vi "ChordsRecognitionFinal.vi"() -> ()   [LabVIEW 2021]
uses:
  <vilib>/Utility/NIReport.llb/Report Type.ctl
  <vilib>/numeric/Random Number (Range) I64.vi
  <vilib>/Analysis/baseanly.llb/Real A x B.vi
  <vilib>/numeric/sub_Random U32.vi
  <vilib>/Utility/file.llb/Read Delimited Spreadsheet (DBL).vi
  <vilib>/addons/_office/excel.llb/Excel Easy Table (str).vi
  <vilib>/Analysis/Matrix/Numeric/Conversions/Matrix To Array - RM.vi
  <vilib>/Utility/NIReport.llb/NI_report.lvclass
  <vilib>/Analysis/NI_AALBase.lvlib
  <vilib>/Analysis/Matrix/NI_Matrix.lvlib
  <vilib>/Utility/NIReport.llb/NI_ReportGenerationCore.lvlib
  <vilib>/Utility/NIReport.llb/Excel/NI_Excel.lvclass
  <vilib>/addons/_office/NI_ReportGenerationToolkit.lvlib
panel:
  in  "Save":bool
  in  "Init":bool
  in  "Aux":dbl
  in  "Saved":bool
  out "n":i32
  in  "Y_ideal":dbl[][][](array[numeric])
  out "Playing":string
  out "Keys":bool[][](array[boolean])
  out "la#":bool
  out "sol#":bool
  out "fa#":bool
  out "re#":bool
  out "do#":bool
  out "si":bool
  out "la":bool
  out "sol":bool
  out "fa":bool
  out "mi":bool
  out "re":bool
  out "do":bool
  out "Confidence":dbl
  out "min value":dbl
  out "max value":dbl
  in  "Init - Random":bool
  in  "Output":i32=1
  in  "2th layer":i32=2
  in  "1th layer":i32=3
  in  "Predict":bool
  out "Error":dbl[](array[numeric])
  in  "W1":dbl[][](array[numeric])
  out "Y":dbl[][](array[numeric])
  in  "Learn?":bool
  in  "Lr":dbl
  in  "?":bool
  in  "Bias 2":dbl[][](array[numeric]) format="%#_13g"
  in  "Bias 3":dbl[][](array[numeric]) format="%#_13g"
  in  "Bias 1":dbl[][](array[numeric]) format="%#_13g"
  in  "W2":dbl[][](array[numeric])
  in  "W3":dbl[][](array[numeric])
  out "C":i16[][](array[numeric])
  in  "index":i32
  out "BoolAux":bool[](array[boolean])
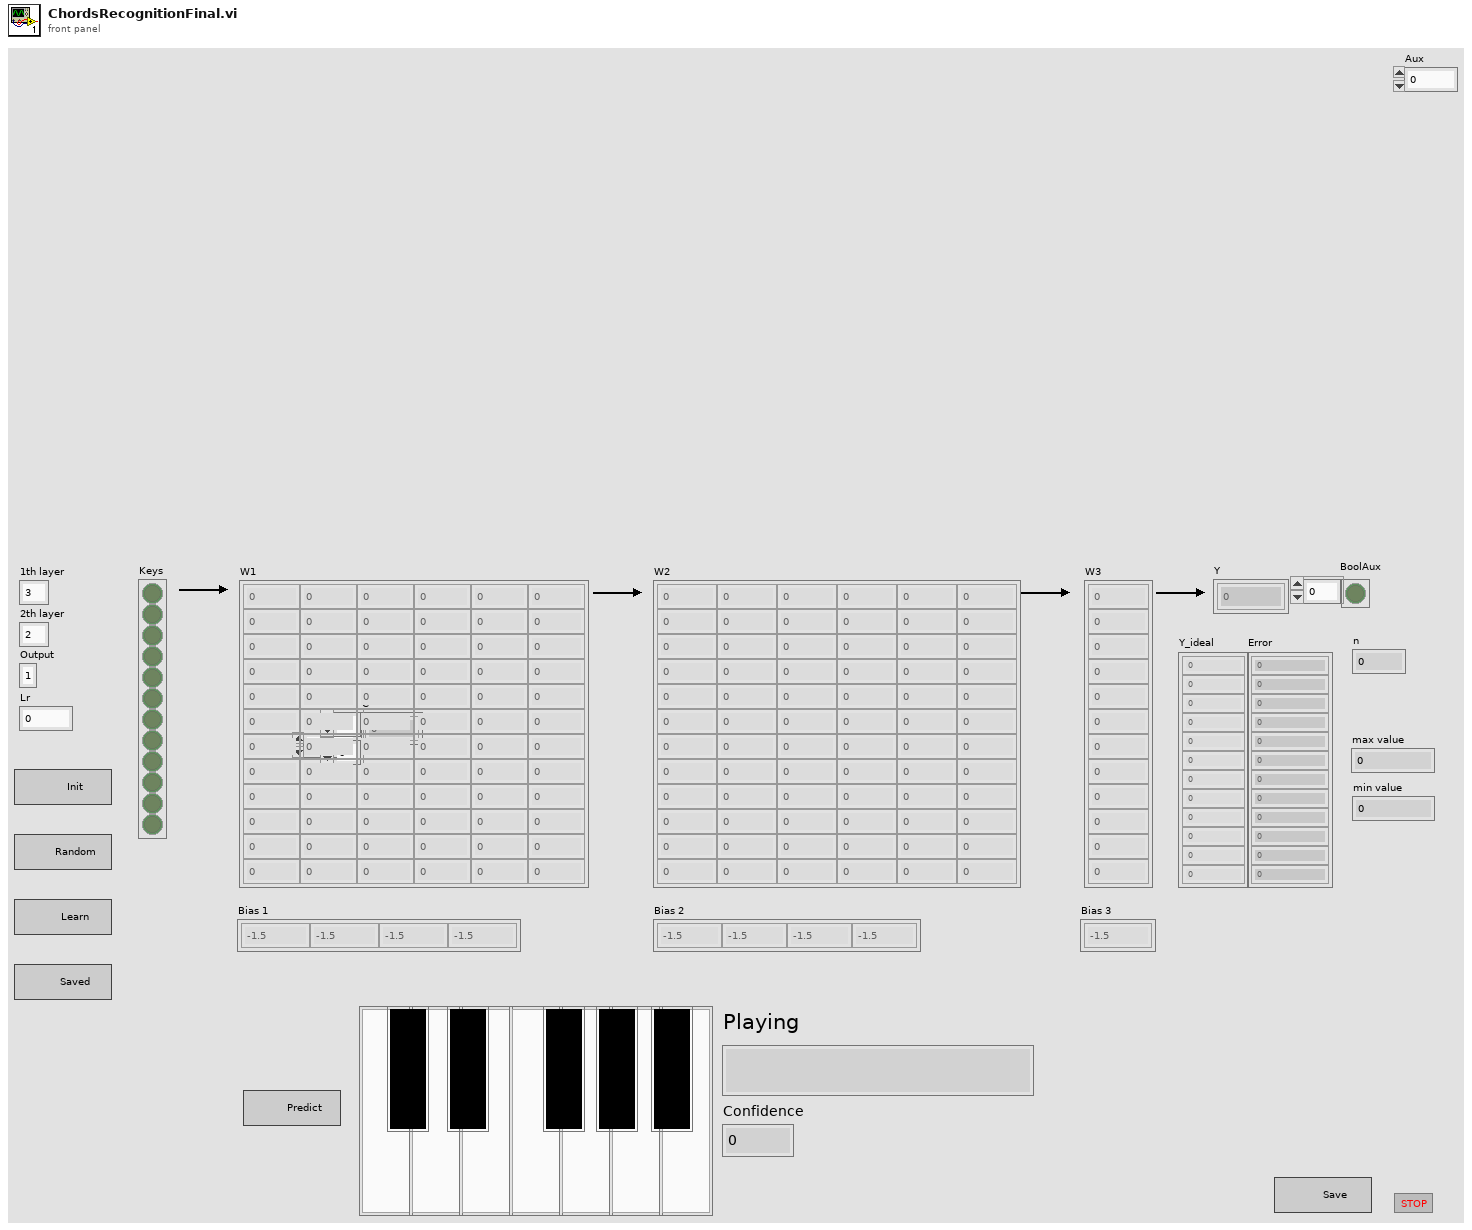
[diagram p1: front panel]
types:
  T1 = typedef "NI_ReportGenerationCore.lvlib/Report Type.ctl" = enum16{"HTML", "Word", "Excel"}
  T2 = typedef "NI_Matrix.lvlib/RealMatrix.ctl" = dbl[][]
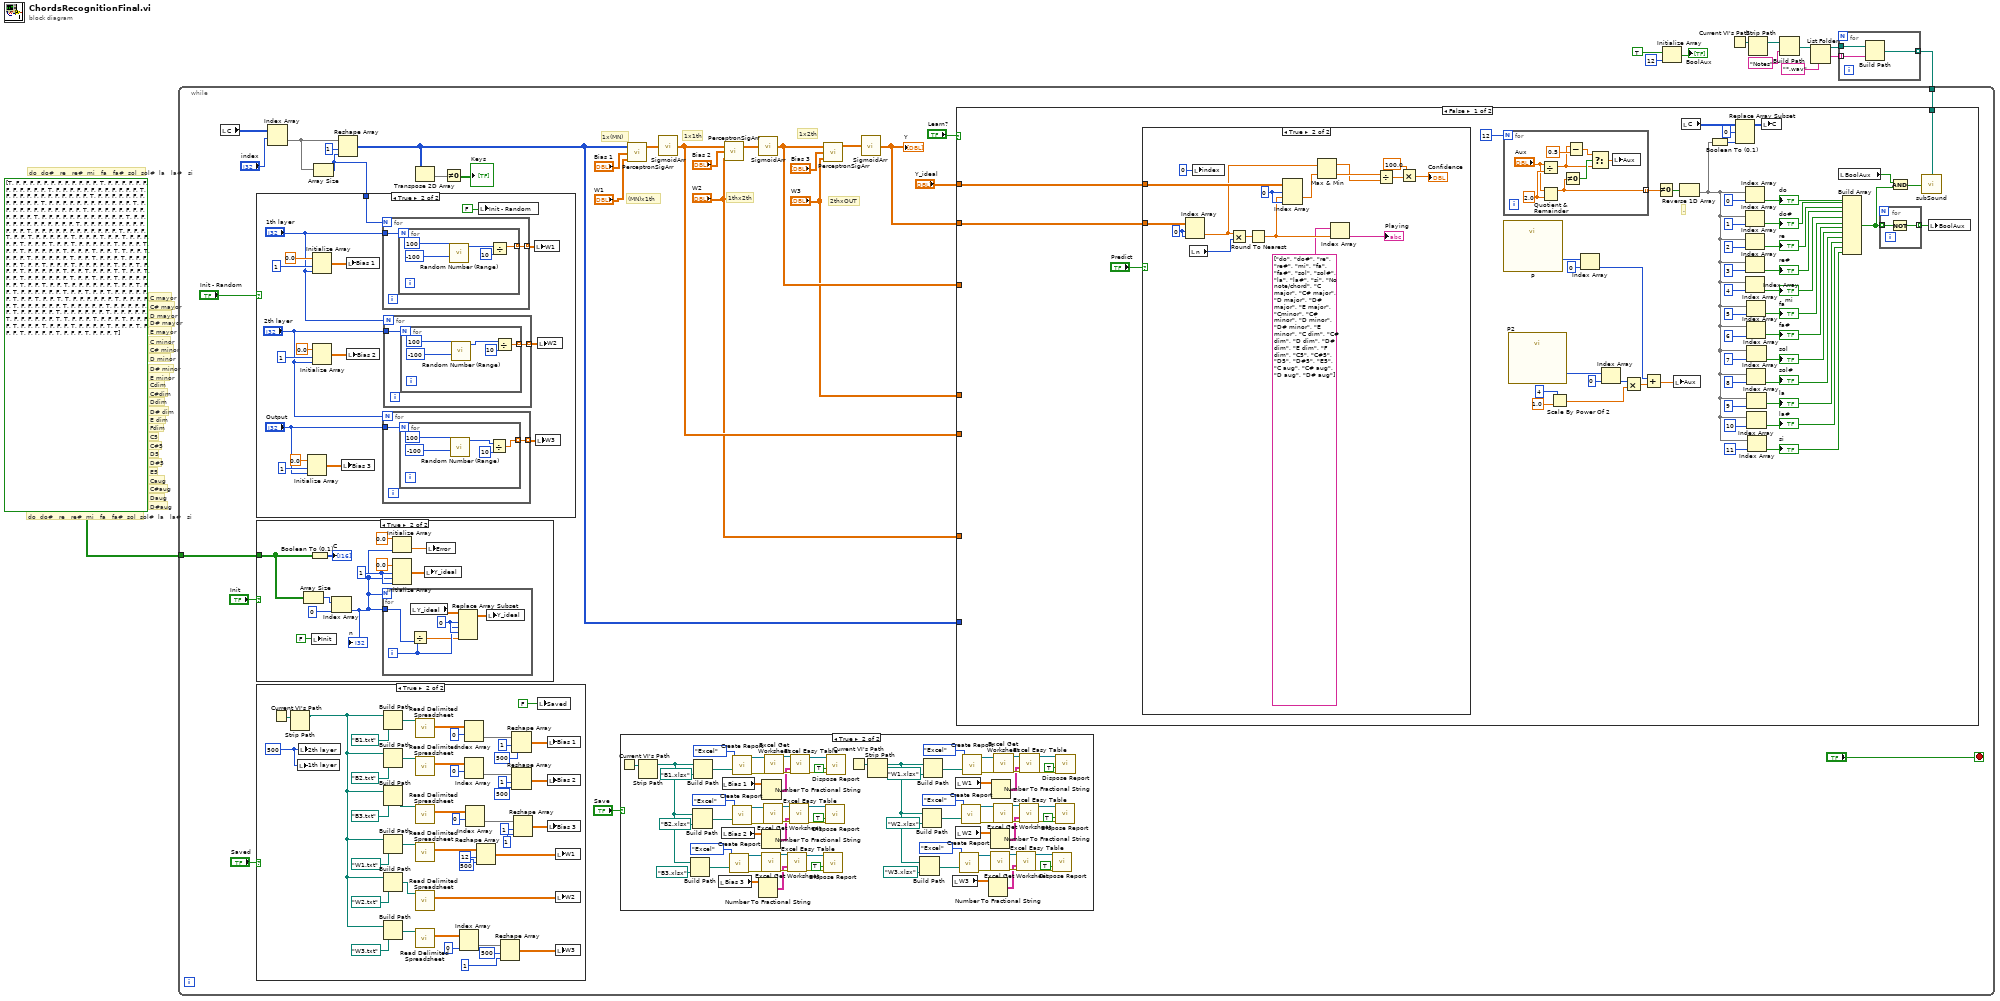
[diagram p0: block diagram]
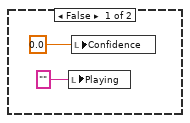
[diagram p6: hidden frame]
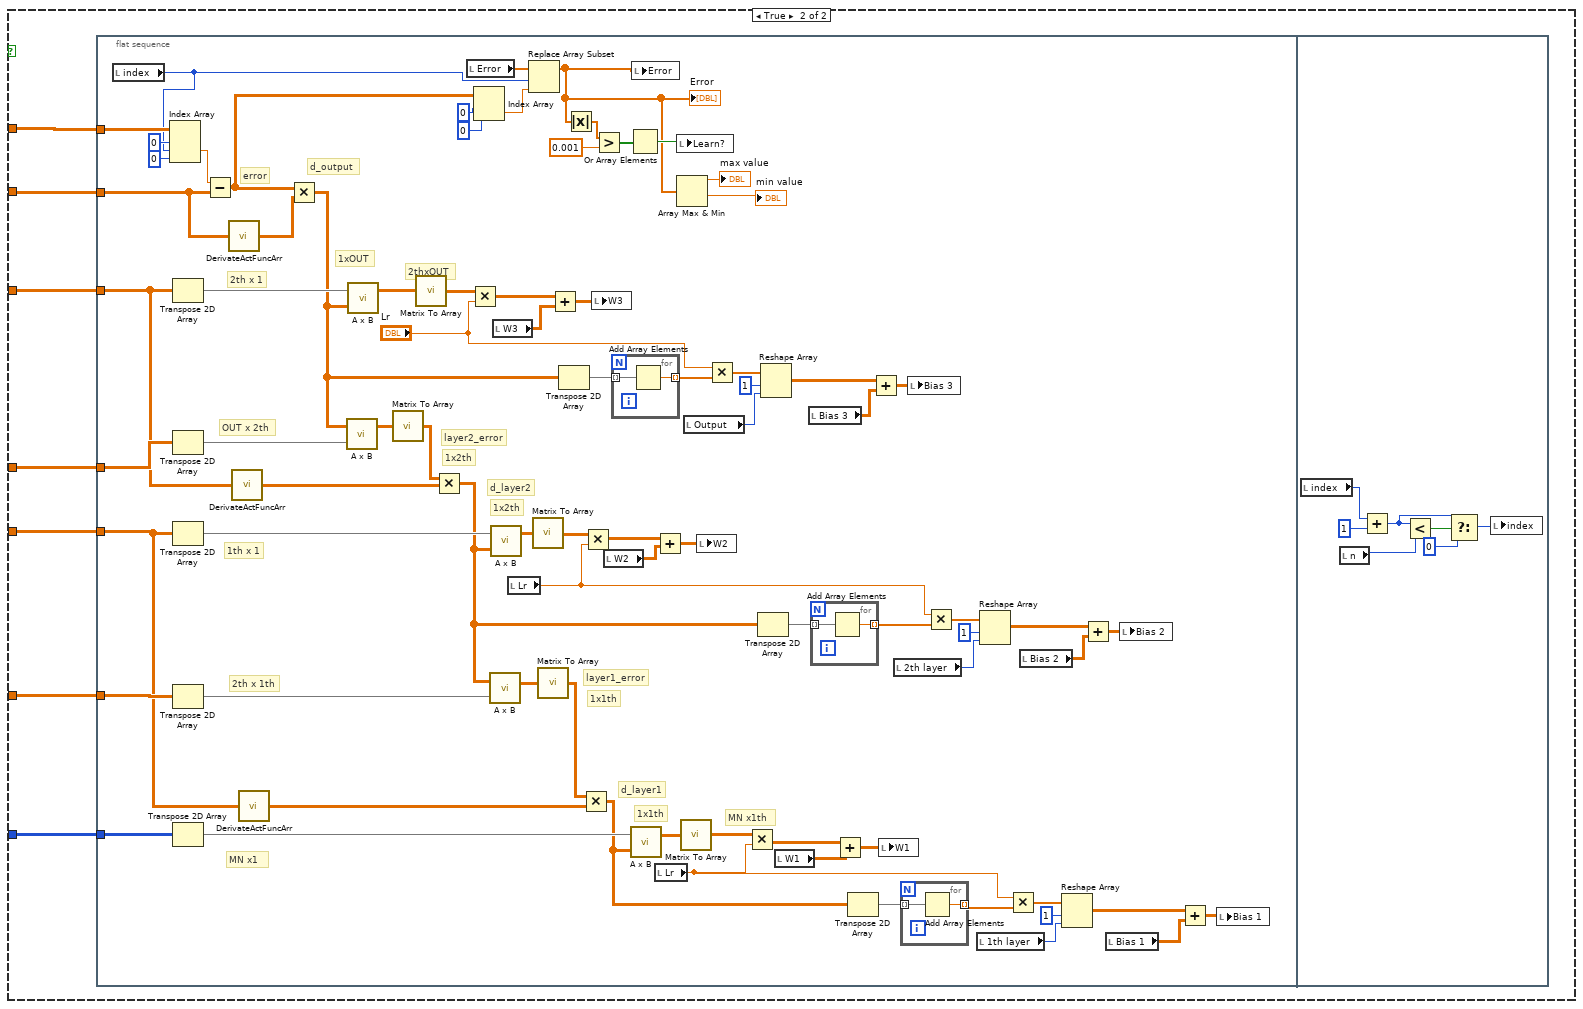
[diagram p7: hidden frame]
diagram:
  # "D#aug"
  # "Daug"
  # "C#aug"
  # "Caug"
  # "D# dim"
  # "D5"
  # "Ddim"
  # "C#5"
  # "C#dim"
  # "C5"
  # "Cdim"
  # "Fdim"
  # "E5"
  # "E dim"
  # "E minor"
  # "E mayor"
  # "D#5"
  # "D# minor"
  # "D# mayor"
  # "D minor"
  # "D mayor"
  # "C# minor"
  # "C# mayor"
  # "C minor"
  # "C mayor"
  # "do  do#   re   re#  mi   fa   fa#  sol  sol#  la   la#   si"
  # "do  do#   re   re#  mi   fa   fa#  sol  sol#  la   la#   si"
  n1 = Initialize Array(TRUE, 12 ("dimension size")) -> (→"BoolAux":bool[])
  n2 = Current VI's Path() -> (path=w8:path)
  n3 = Strip Path(path=w8) -> (stripped path=w9:path)  [unwired: 1 out]
  n4 = Build Path(base path=w9, name or relative path="Notes") -> (appended path=w12:path)
  n5 = List Folder(path=w12, pattern="*.wav") -> (path out=w10:path, filenames=w11:string[])  [unwired: 1 in, 3 out]
  n6 = for {
    tunnel: w10 -> [w15]
    tunnel: w11 -> [w14] mode=indexing
    tunnel: [w13] -> w2 mode=indexing
    n7 = Build Path(base path=w15, name or relative path=w14) -> (appended path=w13:path)
  }
  n8 = while {
    tunnel: w2 -> [w19]
    tunnel: bool[][] [[TRUE, FALSE, FALSE, FALSE, FALSE, FALSE, FALSE, FALSE, FALSE, FALSE, FALSE, FALSE], [FALSE, TRUE, FALSE, FALSE, FALSE, FALSE, FALSE, FALSE, FALSE, FALSE, FALSE, FALSE], [FALSE, FALSE, TRUE, FALSE, FALSE, FALSE, FALSE, FALSE, FALSE, FALSE, FALSE, FALSE], [FALSE, FALSE, FALSE, TRUE, FALSE, FALSE, FALSE, FALSE, FALSE, FALSE, FALSE, FALSE], [FALSE, FALSE, FALSE, FALSE, TRUE, FALSE, FALSE, FALSE, FALSE, FALSE, FALSE, FALSE], [FALSE, FALSE, FALSE, FALSE, FALSE, TRUE, FALSE, FALSE, FALSE, FALSE, FALSE, FALSE], [FALSE, FALSE, FALSE, FALSE, FALSE, FALSE, TRUE, FALSE, FALSE, FALSE, FALSE, FALSE], [FALSE, FALSE, FALSE, FALSE, FALSE, FALSE, FALSE, TRUE, FALSE, FALSE, FALSE, FALSE], [FALSE, FALSE, FALSE, FALSE, FALSE, FALSE, FALSE, FALSE, TRUE, FALSE, FALSE, FALSE], [FALSE, FALSE, FALSE, FALSE, FALSE, FALSE, FALSE, FALSE, FALSE, TRUE, FALSE, FALSE], [FALSE, FALSE, FALSE, FALSE, FALSE, FALSE, FALSE, FALSE, FALSE, FALSE, TRUE, FALSE], [FALSE, FALSE, FALSE, FALSE, FALSE, FALSE, FALSE, FALSE, FALSE, FALSE, FALSE, TRUE], [FALSE, FALSE, FALSE, FALSE, FALSE, FALSE, FALSE, FALSE, FALSE, FALSE, FALSE, FALSE], [TRUE, FALSE, FALSE, FALSE, TRUE, FALSE, FALSE, TRUE, FALSE, FALSE, FALSE, FALSE], [FALSE, TRUE, FALSE, FALSE, FALSE, TRUE, FALSE, FALSE, TRUE, FALSE, FALSE, FALSE], [FALSE, FALSE, TRUE, FALSE, FALSE, FALSE, TRUE, FALSE, FALSE, TRUE, FALSE, FALSE], [FALSE, FALSE, FALSE, TRUE, FALSE, FALSE, FALSE, TRUE, FALSE, FALSE, TRUE, FALSE], [FALSE, FALSE, FALSE, FALSE, TRUE, FALSE, FALSE, FALSE, TRUE, FALSE, FALSE, TRUE], [TRUE, FALSE, FALSE, TRUE, FALSE, FALSE, FALSE, TRUE, FALSE, FALSE, FALSE, FALSE], [FALSE, TRUE, FALSE, FALSE, TRUE, FALSE, FALSE, FALSE, TRUE, FALSE, FALSE, FALSE], [FALSE, FALSE, TRUE, FALSE, FALSE, TRUE, FALSE, FALSE, FALSE, TRUE, FALSE, FALSE], [FALSE, FALSE, FALSE, TRUE, FALSE, FALSE, TRUE, FALSE, FALSE, FALSE, TRUE, FALSE], [FALSE, FALSE, FALSE, FALSE, TRUE, FALSE, FALSE, TRUE, FALSE, FALSE, FALSE, TRUE], [TRUE, FALSE, FALSE, TRUE, FALSE, FALSE, TRUE, FALSE, FALSE, FALSE, FALSE, FALSE], [FALSE, TRUE, FALSE, FALSE, TRUE, FALSE, FALSE, TRUE, FALSE, FALSE, FALSE, FALSE], [FALSE, FALSE, TRUE, FALSE, FALSE, TRUE, FALSE, FALSE, TRUE, FALSE, FALSE, FALSE], [FALSE, FALSE, FALSE, TRUE, FALSE, FALSE, TRUE, FALSE, FALSE, TRUE, FALSE, FALSE], [FALSE, FALSE, FALSE, FALSE, TRUE, FALSE, FALSE, TRUE, FALSE, FALSE, TRUE, FALSE], [FALSE, FALSE, FALSE, FALSE, FALSE, TRUE, FALSE, FALSE, TRUE, FALSE, FALSE, TRUE], [TRUE, FALSE, FALSE, FALSE, FALSE, FALSE, FALSE, TRUE, FALSE, FALSE, FALSE, FALSE], [FALSE, TRUE, FALSE, FALSE, FALSE, FALSE, FALSE, FALSE, TRUE, FALSE, FALSE, FALSE], [FALSE, FALSE, TRUE, FALSE, FALSE, FALSE, FALSE, FALSE, FALSE, TRUE, FALSE, FALSE], [FALSE, FALSE, FALSE, TRUE, FALSE, FALSE, FALSE, FALSE, FALSE, FALSE, TRUE, FALSE], [FALSE, FALSE, FALSE, FALSE, TRUE, FALSE, FALSE, FALSE, FALSE, FALSE, FALSE, TRUE], [TRUE, FALSE, FALSE, FALSE, TRUE, FALSE, FALSE, FALSE, TRUE, FALSE, FALSE, FALSE], [FALSE, TRUE, FALSE, FALSE, FALSE, TRUE, FALSE, FALSE, FALSE, TRUE, FALSE, FALSE], [FALSE, FALSE, TRUE, FALSE, FALSE, FALSE, TRUE, FALSE, FALSE, FALSE, TRUE, FALSE], [FALSE, FALSE, FALSE, TRUE, FALSE, FALSE, FALSE, TRUE, FALSE, FALSE, FALSE, TRUE]] -> [w17]
    stop <- "?" stop-if-true
    # "2thxOUT"
    # "1x2th"
    # "1thx2th"
    # "1x1th"
    # "1x(MN)"
    # "(MN)x1th"
    n9 = local read "C"() -> (w21:i16[][])
    n10 = case shown="True" "Init" {
      tunnel: w17 -> [_ w122]
      frame False {
      }
      frame True {
        w129 = 1 ("dimension size")
        n11 = Array Size(array=w122) -> (size(s)=w124:i32[])
        n12 = Boolean To (0,1)(Boolean=w122) -> (0, 1=→"C":i16[][])
        n13 = local write "Init"(FALSE ("Init")) -> ()
        n14 = Index Array(array=w124, index=0) -> (element=w125:i32)
        "n" <- w125
        n15 = for {
          N: w125 -> [_]
          tunnel: w125 -> [w133]
          i -> [w134]
          w135 = 0 ("index (page)")
          n16 = local read "Y_ideal"() -> (w136:dbl[][][])
          n17 = Divide(x=w134, y=w133) -> (x/y=w132:dbl)
          n18 = Replace Array Subset(array=w136, new element=w132, index (dim 0)=w135, index (dim 1)=w134, index (dim 2)=w135) -> (w137:dbl[][][])
          n19 = local write "Y_ideal"(w137) -> ()
        }
        n20 = Initialize Array(0.0 ("element"), w125) -> (w130:dbl[])
        n21 = Initialize Array(0.0 ("element"), w129, w125, w129) -> (w128:dbl[][][])
        n22 = local write "Y_ideal"(w128) -> ()
        n23 = local write "Error"(w130) -> ()
      }
    }
    n24 = case shown="True" "Saved" {
      frame False {
      }
      frame True {
        w181 = 500 ("1th layer")
        n25 = Current VI's Path() -> (path=w139:path)
        n26 = Strip Path(path=w139) -> (stripped path=w138:path)  [unwired: 1 out]
        n27 = local write "1th layer"(w181) -> ()
        n28 = local write "2th layer"(w181) -> ()
        n29 = Build Path(base path=w138, name or relative path=path "B1.txt") -> (appended path=w159:path)
        n30 = Build Path(base path=w138, name or relative path=path "B2.txt") -> (appended path=w157:path)
        n31 = Build Path(base path=w138, name or relative path=path "B3.txt") -> (appended path=w155:path)
        n32 = Build Path(base path=w138, name or relative path=path "W1.txt") -> (appended path=w153:path)
        n33 = Build Path(base path=w138, name or relative path=path "W2.txt") -> (appended path=w149:path)
        n34 = Build Path(base path=w138, name or relative path=path "W3.txt") -> (appended path=w147:path)
        n35 = call-poly <vilib>:"Read Delimited Spreadsheet.vi"("file path (dialog if empty)"=w159) -> ("all rows"=w180:dbl[][])  [unwired: 9 in, 5 out]
        n36 = call-poly <vilib>:"Read Delimited Spreadsheet.vi"("file path (dialog if empty)"=w157) -> ("all rows"=w172:dbl[][])  [unwired: 9 in, 5 out]
        n37 = call-poly <vilib>:"Read Delimited Spreadsheet.vi"("file path (dialog if empty)"=w155) -> ("all rows"=w152:dbl[][])  [unwired: 9 in, 5 out]
        n38 = call-poly <vilib>:"Read Delimited Spreadsheet.vi"("file path (dialog if empty)"=w153) -> ("all rows"=w151:dbl[][])  [unwired: 9 in, 5 out]
        n39 = call-poly <vilib>:"Read Delimited Spreadsheet.vi"("file path (dialog if empty)"=w149) -> ("all rows"=w141:dbl[][])  [unwired: 9 in, 5 out]
        n40 = call-poly <vilib>:"Read Delimited Spreadsheet.vi"("file path (dialog if empty)"=w147) -> ("all rows"=w146:dbl[][])  [unwired: 9 in, 5 out]
        n41 = Index Array(array=w146, index (col)=0 ("index (row)")) -> (element=w164:dbl[])  [unwired: 1 in]
        n42 = Index Array(array=w180, index (row)=0) -> (element=w178:dbl[])  [unwired: 1 in]
        n43 = Index Array(array=w172, index (row)=0) -> (element=w174:dbl[])  [unwired: 1 in]
        n44 = Index Array(array=w152, index (row)=0) -> (element=w169:dbl[])  [unwired: 1 in]
        n45 = Reshape Array(w151, 12 ("dimension size"), 500 ("dimension size")) -> (w142:dbl[][])
        n46 = Reshape Array(w164, 500 ("dimension size"), 1 ("dimension size")) -> (w140:dbl[][])
        n47 = Reshape Array(w178, 1 ("dimension size"), 500 ("dimension size")) -> (w145:dbl[][])
        n48 = Reshape Array(w174, 1 ("dimension size"), 500 ("dimension size")) -> (w144:dbl[][])
        n49 = Reshape Array(w169, 1 ("dimension size"), 1 ("dimension size")) -> (w143:dbl[][])
        n50 = local write "Saved"(FALSE ("Boolean")) -> ()
        n51 = local write "Bias 1"(w145) -> ()
        n52 = local write "Bias 2"(w144) -> ()
        n53 = local write "Bias 3"(w143) -> ()
        n54 = local write "W1"(w142) -> ()
        n55 = local write "W2"(w141) -> ()
        n56 = local write "W3"(w140) -> ()
      }
    }
    n57 = Index Array(array=w21, index (row)="index") -> (element=w26:i16[])  [unwired: 1 in]
    n58 = Array Size(array=w26) -> (size(s)=w27:i32)
    n59 = case shown="True" "Init - Random" {
      tunnel: w27 -> [_ w198]
      frame False {
      }
      frame True {
        n60 = Initialize Array(0.0 ("element"), 1 ("dimension size"), "Output") -> (w183:dbl[][])
        n61 = Initialize Array(0.0 ("element"), 1 ("dimension size"), "1th layer") -> (w197:dbl[][])
        n62 = Initialize Array(0.0 ("element"), 1 ("dimension size"), "2th layer") -> (w192:dbl[][])
        n63 = local write "Bias 3"(w183) -> ()
        n64 = local write "Bias 1"(w197) -> ()
        n65 = local write "Bias 2"(w192) -> ()
        n66 = for {
          N: w198 -> [_]
          tunnel: "1th layer" -> [w215]
          tunnel: [w214] -> w194 mode=indexing
          n67 = for {
            N: w215 -> [_]
            tunnel: [w217] -> w214 mode=indexing
            n68 = call-poly <vilib>:"Random Number (Range).vi"("lower bound (-100)"=i64 -100, "upper bound (100)"=i64 100) -> ("number"=w218:i64)  [unwired: 9 in]
            n69 = Divide(x=w218, y=i64 10) -> (x/y=w217:dbl)
          }
        }
        n70 = for {
          N: "2th layer" -> [_]
          tunnel: "Output" -> [w201]
          tunnel: [w200] -> w187 mode=indexing
          n71 = for {
            N: w201 -> [_]
            tunnel: [w202] -> w200 mode=indexing
            n72 = call-poly <vilib>:"Random Number (Range).vi"("lower bound (-100)"=i64 -100, "upper bound (100)"=i64 100) -> ("number"=w203:i64)  [unwired: 9 in]
            n73 = Divide(x=w203, y=i64 10) -> (x/y=w202:dbl)
          }
        }
        n74 = for {
          N: "1th layer" -> [_]
          tunnel: "2th layer" -> [w208]
          tunnel: [w207] -> w188 mode=indexing
          n75 = for {
            N: w208 -> [_]
            tunnel: [w210] -> w207 mode=indexing
            n76 = call-poly <vilib>:"Random Number (Range).vi"("lower bound (-100)"=i64 -100, "upper bound (100)"=i64 100) -> ("number"=w209:i64)  [unwired: 9 in]
            n77 = Divide(x=w209, y=i64 10) -> (x/y=w210:dbl)
          }
        }
        n78 = local write "Init - Random"(FALSE ("Init")) -> ()
        n79 = local write "W1"(w194) -> ()
        n80 = local write "W3"(w187) -> ()
        n81 = local write "W2"(w188) -> ()
      }
    }
    n82 = Reshape Array(w26, 1 ("dimension size"), w27) -> (w25:i16[][])
    n83 = Transpose 2D Array(2D array=w25) -> (transposed array=w23:i16[][])
    n84 = Not Equal To 0?(x=w23) -> (x != 0?=→"Keys":bool[][])
    n85 = case shown="True" "Save" {
      frame False {
      }
      frame True {
        n86 = Current VI's Path() -> (path=w120:path)
        n87 = Strip Path(path=w120) -> (stripped path=w45:path)  [unwired: 1 out]
        n88 = Build Path(base path=w45, name or relative path=path "B3.xlsx") -> (appended path=w96:path)
        n89 = Build Path(base path=w45, name or relative path=path "B2.xlsx") -> (appended path=w108:path)
        n90 = Build Path(base path=w45, name or relative path=path "B1.xlsx") -> (appended path=w119:path)
        n91 = local read "Bias 3"() -> (w90:dbl[][])
        n92 = local read "Bias 2"() -> (w102:dbl[][])
        n93 = local read "Bias 1"() -> (w113:dbl[][])
        n94 = call <vilib>:"Create Report.vi"("report type"=Report_Type."Excel", "template (empty)"=w96) -> ("report out"=w94:refnum<class "NI_report.lvclass">, "error out"=w93:errorcluster)  [unwired: 12 in]
        n95 = call <vilib>:"Create Report.vi"("report type"=Report_Type."Excel", "template (empty)"=w108) -> ("report out"=w106:refnum<class "NI_report.lvclass">, "error out"=w105:errorcluster)  [unwired: 12 in]
        n96 = call <vilib>:"Create Report.vi"("report type"=Report_Type."Excel", "template (empty)"=w119) -> ("report out"=w117:refnum<class "NI_report.lvclass">, "error out"=w116:errorcluster)  [unwired: 12 in]
        n97 = Number To Fractional String(number=w90) -> (F-format string=w89:string[][])  [unwired: 3 in]
        n98 = Number To Fractional String(number=w102) -> (F-format string=w101:string[][])  [unwired: 3 in]
        n99 = call <vilib>:"Excel Get Worksheet.vi"("report in"=w94, "error in (no error)"=w93) -> ("report out"=w92:refnum<class "NI_report.lvclass">, "error out"=w91:errorcluster)  [unwired: 12 in]
        n100 = Number To Fractional String(number=w113) -> (F-format string=w112:string[][])  [unwired: 3 in]
        n101 = call <vilib>:"Excel Get Worksheet.vi"("report in"=w106, "error in (no error)"=w105) -> ("report out"=w104:refnum<class "NI_report.lvclass">, "error out"=w103:errorcluster)  [unwired: 12 in]
        n102 = call <vilib>:"Excel Get Worksheet.vi"("report in"=w117, "error in (no error)"=w116) -> ("report out"=w115:refnum<class "NI_report.lvclass">, "error out"=w114:errorcluster)  [unwired: 12 in]
        n103 = call-poly <vilib>:"Excel Easy Table.vi"("report in"=w92, "text data"=w89, "error in (no error)"=w91) -> ("report out"=w88:refnum<class "NI_report.lvclass">, "error out"=w87:errorcluster)  [unwired: 8 in, 3 out]
        n104 = call-poly <vilib>:"Excel Easy Table.vi"("report in"=w104, "text data"=w101, "error in (no error)"=w103) -> ("report out"=w100:refnum<class "NI_report.lvclass">, "error out"=w99:errorcluster)  [unwired: 8 in, 3 out]
        n105 = call-poly <vilib>:"Excel Easy Table.vi"("report in"=w115, "text data"=w112, "error in (no error)"=w114) -> ("report out"=w111:refnum<class "NI_report.lvclass">, "error out"=w110:errorcluster)  [unwired: 8 in, 3 out]
        n106 = call-dynamic "Dispose Report.vi"("report in"=w88, "save changes? (F)"=TRUE, "error in (no error)"=w87) -> ()  [unwired: 12 in, 1 out]
        n107 = call-dynamic "Dispose Report.vi"("report in"=w100, "save changes? (F)"=TRUE, "error in (no error)"=w99) -> ()  [unwired: 12 in, 1 out]
        n108 = call-dynamic "Dispose Report.vi"("report in"=w111, "save changes? (F)"=TRUE, "error in (no error)"=w110) -> ()  [unwired: 12 in, 1 out]
        n109 = Current VI's Path() -> (path=w84:path)
        n110 = Strip Path(path=w84) -> (stripped path=w47:path)  [unwired: 1 out]
        n111 = Build Path(base path=w47, name or relative path=path "W3.xlsx") -> (appended path=w59:path)
        n112 = Build Path(base path=w47, name or relative path=path "W2.xlsx") -> (appended path=w71:path)
        n113 = Build Path(base path=w47, name or relative path=path "W1.xlsx") -> (appended path=w83:path)
        n114 = local read "W3"() -> (w53:dbl[][])
        n115 = local read "W2"() -> (w65:dbl[][])
        n116 = local read "W1"() -> (w77:dbl[][])
        n117 = call <vilib>:"Create Report.vi"("report type"=Report_Type."Excel", "template (empty)"=w59) -> ("report out"=w57:refnum<class "NI_report.lvclass">, "error out"=w56:errorcluster)  [unwired: 12 in]
        n118 = call <vilib>:"Create Report.vi"("report type"=Report_Type."Excel", "template (empty)"=w71) -> ("report out"=w69:refnum<class "NI_report.lvclass">, "error out"=w68:errorcluster)  [unwired: 12 in]
        n119 = call <vilib>:"Create Report.vi"("report type"=Report_Type."Excel", "template (empty)"=w83) -> ("report out"=w81:refnum<class "NI_report.lvclass">, "error out"=w80:errorcluster)  [unwired: 12 in]
        n120 = Number To Fractional String(number=w53) -> (F-format string=w52:string[][])  [unwired: 3 in]
        n121 = Number To Fractional String(number=w65) -> (F-format string=w64:string[][])  [unwired: 3 in]
        n122 = call <vilib>:"Excel Get Worksheet.vi"("report in"=w57, "error in (no error)"=w56) -> ("report out"=w55:refnum<class "NI_report.lvclass">, "error out"=w54:errorcluster)  [unwired: 12 in]
        n123 = Number To Fractional String(number=w77) -> (F-format string=w76:string[][])  [unwired: 3 in]
        n124 = call <vilib>:"Excel Get Worksheet.vi"("report in"=w69, "error in (no error)"=w68) -> ("report out"=w67:refnum<class "NI_report.lvclass">, "error out"=w66:errorcluster)  [unwired: 12 in]
        n125 = call <vilib>:"Excel Get Worksheet.vi"("report in"=w81, "error in (no error)"=w80) -> ("report out"=w79:refnum<class "NI_report.lvclass">, "error out"=w78:errorcluster)  [unwired: 12 in]
        n126 = call-poly <vilib>:"Excel Easy Table.vi"("report in"=w55, "text data"=w52, "error in (no error)"=w54) -> ("report out"=w51:refnum<class "NI_report.lvclass">, "error out"=w50:errorcluster)  [unwired: 8 in, 3 out]
        n127 = call-poly <vilib>:"Excel Easy Table.vi"("report in"=w67, "text data"=w64, "error in (no error)"=w66) -> ("report out"=w63:refnum<class "NI_report.lvclass">, "error out"=w62:errorcluster)  [unwired: 8 in, 3 out]
        n128 = call-poly <vilib>:"Excel Easy Table.vi"("report in"=w79, "text data"=w76, "error in (no error)"=w78) -> ("report out"=w75:refnum<class "NI_report.lvclass">, "error out"=w74:errorcluster)  [unwired: 8 in, 3 out]
        n129 = call-dynamic "Dispose Report.vi"("report in"=w51, "save changes? (F)"=TRUE, "error in (no error)"=w50) -> ()  [unwired: 12 in, 1 out]
        n130 = call-dynamic "Dispose Report.vi"("report in"=w63, "save changes? (F)"=TRUE, "error in (no error)"=w62) -> ()  [unwired: 12 in, 1 out]
        n131 = call-dynamic "Dispose Report.vi"("report in"=w75, "save changes? (F)"=TRUE, "error in (no error)"=w74) -> ()  [unwired: 12 in, 1 out]
      }
    }
    n132 = call "PerceptronSigArr.vi"("Wa"="W1", "Bias"="Bias 1", "Xa"=w25) -> ("Y"=w38:dbl[][])
    n133 = call "SigmoidArr.vi"("x"=w38) -> ("Sigmoid"=w35:dbl[][])
    n134 = call "PerceptronSigArr.vi"("Wa"="W2", "Bias"="Bias 2", "Xa"=w35) -> ("Y"=w42:dbl[][])
    n135 = call "SigmoidArr.vi"("x"=w42) -> ("Sigmoid"=w33:dbl[][])
    n136 = call "PerceptronSigArr.vi"("Wa"="W3", "Bias"="Bias 3", "Xa"=w33) -> ("Y"=w40:dbl[][])
    n137 = call "SigmoidArr.vi"("x"=w40) -> ("Sigmoid"=w31:dbl[][])
    "Y" <- w31
    n138 = case shown="False" "Learn?" {
      tunnel: w31 -> [w270 w306]
      tunnel: "Y_ideal" -> [w269 w307]
      tunnel: w33 -> [_ w304]
      tunnel: "W3" -> [_ w305]
      tunnel: w35 -> [_ w302]
      tunnel: "W2" -> [_ w303]
      tunnel: w25 -> [_ w301]
      tunnel: w19 -> [w233 _]
      frame False {
        # "."
        n139 = case shown="True" "Predict" {
          tunnel: w270 -> [_ w299]
          tunnel: w269 -> [_ w298]
          frame False {
            n140 = local write "Playing"("" ("Playing")) -> ()
            n141 = local write "Confidence"(0.0 ("Pattern")) -> ()
          }
          frame True {
            w297 = 0 ("disabled index (page)")
            w300 = 0 ("index (row)")
            n142 = Index Array(array=w299, index (row)=w300, index (col)=w300) -> (element=w289:dbl)
            n143 = local read "n"() -> (w287:i32)
            n144 = local write "index"(0 ("index")) -> ()
            n145 = Multiply(x=w289, y=w287) -> (x*y=w293:dbl)
            n146 = Round To Nearest(number=w293) -> (nearest integer value=w286:dbl)
            n147 = Index Array(array=w298, index (dim 0)=w297, index (dim 1)=w286, index (dim 2)=w297) -> (element=w290:dbl)
            n148 = Max & Min(x=w289, y=w290) -> (max(x,y)=w291:dbl, min(x,y)=w292:dbl)
            n149 = Index Array(array=string[] ["do", "do#", "re", "re#", "mi", "fa", "fa#", "sol", "sol#", "la", "la#", "si", "No note/chord", "C major", "C# major", "D major", "D# major", "E major", "Cminor", "C# minor", "D minor", "D# minor", "E minor", "C dim", "C# dim", "D dim", "D# dim", "E dim", "F dim", "C5", "C#5", "D5", "D#5", "E5", "C aug", "C# aug", "D aug", "D# aug"], index=w286) -> (element=→"Playing":string)
            n150 = Divide(x=w292, y=w291) -> (x/y=w296:dbl)
            n151 = Multiply(x=100.0, y=w296) -> (x*y=→"Confidence":dbl)
          }
        }
        n152 = for {
          N: 12 -> [_]
          tunnel: [w280] -> w239 mode=indexing
          w281 = 2.0 ("y")
          n153 = Divide(x="Aux", y=w281) -> (x/y=w277:dbl)
          n154 = Quotient & Remainder(x="Aux", y=w281) -> (x-y*floor(x/y)=w280:dbl)  [unwired: 1 out]
          n155 = Not Equal To 0?(x=w280) -> (x != 0?=w279:bool)
          n156 = Subtract(x=w277, y=0.5) -> (x-y=w276:dbl)
          n157 = Select(t=w276, s=w279, f=w277) -> (s? t:f=w275:dbl)
          n158 = local write "Aux"(w275) -> ()
        }
        n159 = call "P"() -> ("data"=w250:u32[])  [unwired: 17 in, 2 out]
        n160 = call "P2"() -> ("data"=w248:u32[])  [unwired: 17 in, 2 out]
        n161 = Scale By Power Of 2(n=i16 4, x=1.0) -> (x*2^n=w244:dbl)
        n162 = Index Array(array=w250, index=0) -> (element=w242:u32)
        n163 = Index Array(array=w248, index=0) -> (element=w247:u32)
        n164 = Multiply(x=w247, y=w244) -> (x*y=w243:dbl)
        n165 = Add(x=w242, y=w243) -> (x+y=w241:dbl)
        n166 = Not Equal To 0?(x=w239) -> (x != 0?=w240:bool[])
        n167 = local write "Aux"(w241) -> ()
        n168 = Reverse 1D Array(array=w240) -> (reversed array=w238:bool[])
        n169 = local read "C"() -> (w267:i16[][])
        n170 = Boolean To (0,1)(Boolean=w238) -> (0, 1=w266:i16[])
        n171 = Replace Array Subset(array=w267, new element=w266, index (row)=0) -> (w268:i16[][])  [unwired: 1 in]
        n172 = Index Array(array=w238, index=0) -> (element=w232:bool)
        "do" <- w232
        n173 = Index Array(array=w238, index=2) -> (element=w230:bool)
        "re" <- w230
        n174 = Index Array(array=w238, index=1) -> (element=w231:bool)
        "do#" <- w231
        n175 = Index Array(array=w238, index=3) -> (element=w229:bool)
        "re#" <- w229
        n176 = Index Array(array=w238, index=4) -> (element=w228:bool)
        "mi" <- w228
        n177 = Index Array(array=w238, index=5) -> (element=w227:bool)
        "fa" <- w227
        n178 = Index Array(array=w238, index=6) -> (element=w226:bool)
        "fa#" <- w226
        n179 = Index Array(array=w238, index=8) -> (element=w224:bool)
        "sol#" <- w224
        n180 = Index Array(array=w238, index=7) -> (element=w225:bool)
        "sol" <- w225
        n181 = Index Array(array=w238, index=9) -> (element=w223:bool)
        "la" <- w223
        n182 = Index Array(array=w238, index=10) -> (element=w222:bool)
        "la#" <- w222
        n183 = Index Array(array=w238, index=11) -> (element=w221:bool)
        "si" <- w221
        n184 = local write "C"(w268) -> ()
        n185 = local read "BoolAux"() -> (w235:bool[])
        n186 = Build Array(w232, w231, w230, w229, w228, w227, w226, w225, w224, w223, w222, w221) -> (w234:bool[])
        n187 = for {
          tunnel: w234 -> [w273] mode=indexing
          tunnel: [w272] -> w237 mode=indexing
          n188 = Not(x=w273) -> (.not. x?=w272:bool)
        }
        n189 = And(x=w235, y=w234) -> (x .and. y?=w236:bool[])
        n190 = call "subSound.vi"("Array 2"=w233, "Array"=w236) -> ()
        n191 = local write "BoolAux"(w237) -> ()
      }
      frame True {
        n192 = flat-sequence {
          tunnel: w307 -> [w324]
          tunnel: w306 -> [w375]
          tunnel: w305 -> [w363]
          tunnel: w304 -> [w360]
          tunnel: w303 -> [w346]
          tunnel: w302 -> [w342]
          tunnel: w301 -> [w328]
          frame #0 {
            # "MN x1th"
            # "MN x1"
            # "1x1th"
            # "d_layer1"
            # "1x1th"
            # "layer1_error"
            # "2th x 1th"
            # "1th x 1"
            # "1x2th"
            # "OUT x 2th"
            # "d_layer2"
            # "1x2th"
            # "layer2_error"
            # "2thxOUT"
            # "1xOUT"
            # "2th x 1"
            # "d_output"
            # "error"
            n193 = local read "index"() -> (w320:i32)
            n194 = Index Array(array=w324, index (dim 0)=0 ("index (page)"), index (dim 1)=w320, index (dim 2)=0 ("disabled index (col)")) -> (element=w323:dbl)
            n195 = Transpose 2D Array(2D array=w360) -> (transposed array=w373:dbl[][])
            n196 = Transpose 2D Array(2D array=w363) -> (transposed array=w362:dbl[][])
            n197 = Transpose 2D Array(2D array=w342) -> (transposed array=w357:dbl[][])
            n198 = Transpose 2D Array(2D array=w346) -> (transposed array=w345:dbl[][])
            n199 = Transpose 2D Array(2D array=w328) -> (transposed array=w340:i16[][])
            n200 = Subtract(x=w323, y=w375) -> (x-y=w315:dbl[][])
            n201 = call "DerivateActFuncArr.vi"("Input"=w375) -> ("Output"=w374:dbl[][])
            n202 = call "DerivateActFuncArr.vi"("Input"=w360) -> ("Output"=w361:dbl[][])
            n203 = call "DerivateActFuncArr.vi"("Input"=w342) -> ("Output"=w341:dbl[][])
            n204 = Multiply(x=w315, y=w374) -> (x*y=w327:dbl[][])
            n205 = call-poly <vilib>:"A x B.vi"("B"=w362, "A"=w327) -> ("A x B"=w359:T2)  [unwired: 1 out]
            n206 = call-poly <vilib>:"A x B.vi"("B"=w327, "A"=w373) -> ("A x B"=w372:T2)  [unwired: 1 out]
            n207 = call-poly <vilib>:"Matrix To Array.vi"("Real Matrix"=w359) -> ("Real 2D Array"=w358:dbl[][])
            n208 = call-poly <vilib>:"Matrix To Array.vi"("Real Matrix"=w372) -> ("Real 2D Array"=w371:dbl[][])
            n209 = Multiply ("Multiply.vi")(x=w358, y=w361) -> (x*y=w347:dbl[][])
            n210 = local read "Error"() -> (w326:dbl[])
            n211 = Multiply ("Multiply.vi")(x=w371, y="Lr") -> (x*y=w370:dbl[][])
            n212 = Index Array(array=w315, index (row)=0 ("index"), index (col)=0 ("disabled index (col)")) -> (element=w316:dbl)
            n213 = call-poly <vilib>:"A x B.vi"("B"=w345, "A"=w347) -> ("A x B"=w344:T2)  [unwired: 1 out]
            n214 = call-poly <vilib>:"A x B.vi"("B"=w347, "A"=w357) -> ("A x B"=w356:T2)  [unwired: 1 out]
            n215 = local read "W3"() -> (w385:dbl[][])
            n216 = local read "Lr"() -> (w318:dbl)
            n217 = Replace Array Subset(array=w326, new element=w316, index=w320) -> (w311:dbl[])
            "Error" <- w311
            n218 = call-poly <vilib>:"Matrix To Array.vi"("Real Matrix"=w356) -> ("Real 2D Array"=w355:dbl[][])
            n219 = call-poly <vilib>:"Matrix To Array.vi"("Real Matrix"=w344) -> ("Real 2D Array"=w343:dbl[][])
            n220 = Add ("Add.vi")(x=w370, y=w385) -> (x+y=w384:dbl[][])
            n221 = Transpose 2D Array(2D array=w327) -> (transposed array=w369:dbl[][])
            n222 = Absolute Value(x=w311) -> (abs(x)=w309:dbl[])
            n223 = Multiply ("Multiply.vi")(x=w343, y=w341) -> (x*y=w335:dbl[][])
            n224 = Multiply ("Multiply.vi")(x=w355, y=w318) -> (x*y=w354:dbl[][])
            n225 = local write "W3"(w384) -> ()
            n226 = Greater?(x=w309, y=0.001) -> (0:w308:bool[])
            n227 = local read "W2"() -> (w380:dbl[][])
            n228 = for {
              tunnel: w369 -> [w393] mode=indexing
              tunnel: [w392] -> w368 mode=indexing
              n229 = Add Array Elements(numeric array=w393) -> (sum=w392:dbl)
            }
            n230 = Or Array Elements(Boolean array=w308) -> (logical OR=w325:bool)
            n231 = call-poly <vilib>:"A x B.vi"("B"=w335, "A"=w340) -> ("A x B"=w339:T2)  [unwired: 1 out]
            n232 = local write "Error"(w311) -> ()
            n233 = Add ("Add.vi")(x=w354, y=w380) -> (x+y=w381:dbl[][])
            n234 = local read "Lr"() -> (w331:dbl)
            n235 = local write "Learn?"(w325) -> ()
            n236 = Array Max & Min(array=w311) -> (max value=→"max value":dbl, min value=→"min value":dbl)  [unwired: 2 out]
            n237 = call-poly <vilib>:"Matrix To Array.vi"("Real Matrix"=w339) -> ("Real 2D Array"=w338:dbl[][])
            n238 = local read "Output"() -> (w365:i32)
            n239 = local write "W2"(w381) -> ()
            n240 = Multiply ("Multiply.vi")(x="Lr", y=w368) -> (x*y=w367:dbl[])
            n241 = Multiply ("Multiply.vi")(x=w338, y=w331) -> (x*y=w337:dbl[][])
            n242 = Transpose 2D Array(2D array=w347) -> (transposed array=w353:dbl[][])
            n243 = Reshape Array(w367, 1 ("dimension size"), w365) -> (w364:dbl[][])
            n244 = local read "W1"() -> (w387:dbl[][])
            n245 = local read "Bias 3"() -> (w383:dbl[][])
            n246 = for {
              tunnel: w353 -> [w391] mode=indexing
              tunnel: [w390] -> w349 mode=indexing
              n247 = Add Array Elements(numeric array=w391) -> (sum=w390:dbl)
            }
            n248 = Add(x=w337, y=w387) -> (x+y=w386:dbl[][])
            n249 = Transpose 2D Array(2D array=w335) -> (transposed array=w336:dbl[][])
            n250 = Add(x=w364, y=w383) -> (x+y=w382:dbl[][])
            n251 = local write "W1"(w386) -> ()
            n252 = local read "2th layer"() -> (w350:i32)
            n253 = for {
              tunnel: w336 -> [w389] mode=indexing
              tunnel: [w388] -> w332 mode=indexing
              n254 = Add Array Elements(numeric array=w389) -> (sum=w388:dbl)
            }
            n255 = local write "Bias 3"(w382) -> ()
            n256 = Multiply ("Multiply.vi")(x=w318, y=w349) -> (x*y=w352:dbl[])
            n257 = local read "1th layer"() -> (w330:i32)
            n258 = Reshape Array(w352, 1 ("dimension size"), w350) -> (w348:dbl[][])
            n259 = Multiply ("Multiply.vi")(x=w331, y=w332) -> (x*y=w334:dbl[])
            n260 = local read "Bias 2"() -> (w379:dbl[][])
            n261 = Reshape Array(w334, 1 ("dimension size"), w330) -> (w329:dbl[][])
            n262 = Add(x=w348, y=w379) -> (x+y=w378:dbl[][])
            n263 = local read "Bias 1"() -> (w377:dbl[][])
            n264 = local write "Bias 2"(w378) -> ()
            n265 = Add(x=w329, y=w377) -> (x+y=w376:dbl[][])
            n266 = local write "Bias 1"(w376) -> ()
          }
          frame #1 {
            n267 = local read "index"() -> (w396:i32)
            n268 = local read "n"() -> (w394:i32)
            n269 = Add(x=w396, y=1) -> (x+y=w398:i32)
            n270 = Less?(x=w398, y=w394) -> (x < y?=w399:bool)
            n271 = Select(t=w398, s=w399, f=0) -> (s? t:f=w395:i32)
            n272 = local write "index"(w395) -> ()
          }
        }
      }
    }
  }
